vi "te.vi"() -> ()   [LabVIEW 2018]
uses:
  te_state.ctl
  Epimedia_Connex_Source/Controls/Enums/LogLoopEnum.ctl
  Epimedia_Connex_Source/Controls/Clusts/TE_Data_Clust.ctl
panel:
  out "ElapsedRead":u32
  out "Error Out":errorcluster
  out "Enum":T1
  out "Read Progress":dbl(slide) scale=0.0..1.0
  out "On? 3":dbl format="%#.0g"
  out "P 3":dbl format="%.2g"
  out "I 3":dbl format="%.2g"
  out "D 3":dbl format="%.2g"
  out "Set Point 3":dbl format="%.2g"
  out "Temp 3":dbl format="%.2g"
  out "Output 3":dbl format="%.2f"
  out "Polarity 3":dbl format="%#_1g"
  out "Control Type 3":dbl format="%#_1g"
  out "On? 2":dbl format="%#.0g"
  out "P 2":dbl format="%.2g"
  out "I 2":dbl format="%.2g"
  out "D 2":dbl format="%.2g"
  out "Set Point 2":dbl format="%.2g"
  out "Temp 2":dbl format="%.2g"
  out "Output 2":dbl format="%.2f"
  out "Polarity 2":dbl format="%#_1g"
  out "Control Type 2":dbl format="%#_1g"
  out "On?":dbl format="%#.0g"
  out "P 4":dbl format="%.2g"
  out "I 4":dbl format="%.2g"
  out "D 4":dbl format="%.2g"
  out "Set Point 4":dbl format="%.2g"
  out "Temp":dbl format="%.2g"
  out "Output":dbl format="%.2f"
  out "Polarity 4":dbl format="%#_1g"
  out "Control Type 4":dbl format="%#_1g"
  in  "On?":i32 min=0 max=1 format="%_1f"
  in  "P":dbl=5.0 format="%.2g"
  in  "I":dbl format="%.2g"
  in  "D":dbl format="%.2g"
  in  "Set Point":dbl=40.0 format="%.2g"
  in  "Control Type":i32=1 min=0 max=2 format="%_1f"
  in  "Polarity":i32 min=0 max=1 format="%_1f"
  in  "WriteAddressSelect":enum32{"Air", "Bottom Plate ", "Front Plate"}(radio)
  out "Header":picture
  in  "Address":string[](array[string])=["01", "02", "03"]
  in  "Port":refnum<visa-resource-name>="Port1"
  in  "Save Parameters":bool
  out "LED":bool
  in  "stop":bool
  out "Error Dialog":string="Error Message Display Box"
  out "Waveform Chart":cluster{"[0]":dbl, "[0]":dbl, "[0]":dbl}(graph)
  # "°C"
  # "Temp."
  # "%"
  # "Output"
  # "°C"
  # "Control Type:"
  # "0   Deadband\n1   PID\n2   Computer"
  # "Polarity:"
  # "0   HEAT WP1+ and WP2-\n1   HEAT WP2+ and WP1-"
  # "Original Creator: \nMike Zemba, NASA Glenn Research Center\nmichael.j.zemba@nasa.gov\nModified by:\nLuke Graham, Epimedia, Inc.\nluke@epimedia.com"
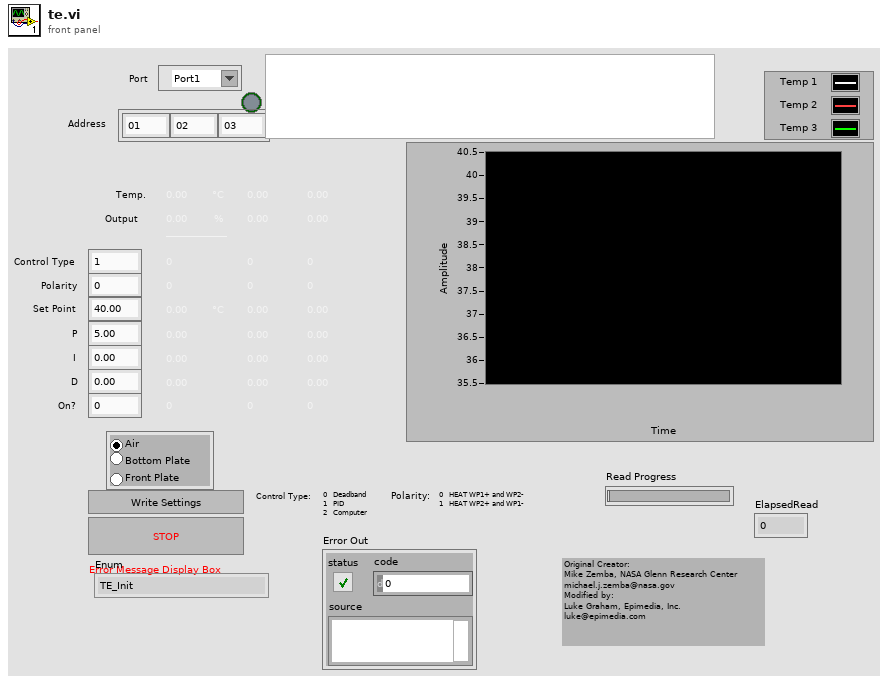
[diagram p1: front panel]
types:
  T1 = typedef "te_state.ctl" = enum16{"TE_Init", "TE_Autotune", "TE_Wait", "TE_Read", "TE_Display", "TE_Send", "TE_Write"}
  T2 = cluster{"port":refnum<visa-resource-name>, "timeout":u32, "baud":u32, "dataBits":u16, "stopBits":u16, "flowControl":u16, "parity":u16, "termChar":bool, "checkSum":bool, "checkSumVal":string}
  T3 = typedef "te_state.ctl" = enum16{"Config", "Autotune", "Wait", "Read", "Log"}
  T4 = typedef "TE_Data_Clust.ctl" = cluster{"TimeString":string, "TimeStamp":dbl, "Temp":dbl, "Output":dbl, "Temp 2":dbl, "Output 2":dbl, "Temp 3":dbl, "Output 3":dbl}
  T5 = typedef "LogLoopEnum.ctl" = enum16{"Log_Init", "Log_Config", "Log_CfgAlarm", "Log_TimeDomain", "Log_Tone", "Log_NoiseTrace", "Log_NoiseSum", "Log_DO", "Log_AI", "Log_TC", "Log_Disdrom", "Log_Weather", "Log_TE", "Log_ADAM", "Log_UPS", "Log_ChkTime", "Log_Alarm", "Log_Write", "Log_Exit"}
  T6 = typedef "imagedata.ctl" = cluster{"image type":i32, "image depth":i32, "image":u8[], "mask":u8[], "colors":u32[], "Rectangle":cluster{"left":i16, "top":i16, "right":i16, "bottom":i16}}
  T7 = cluster{"[0]":dbl, "[1]":dbl, "[2]":dbl, "[3]":dbl, "[4]":dbl, "[5]":dbl, "[6]":dbl, "[7]":dbl, "[8]":dbl}
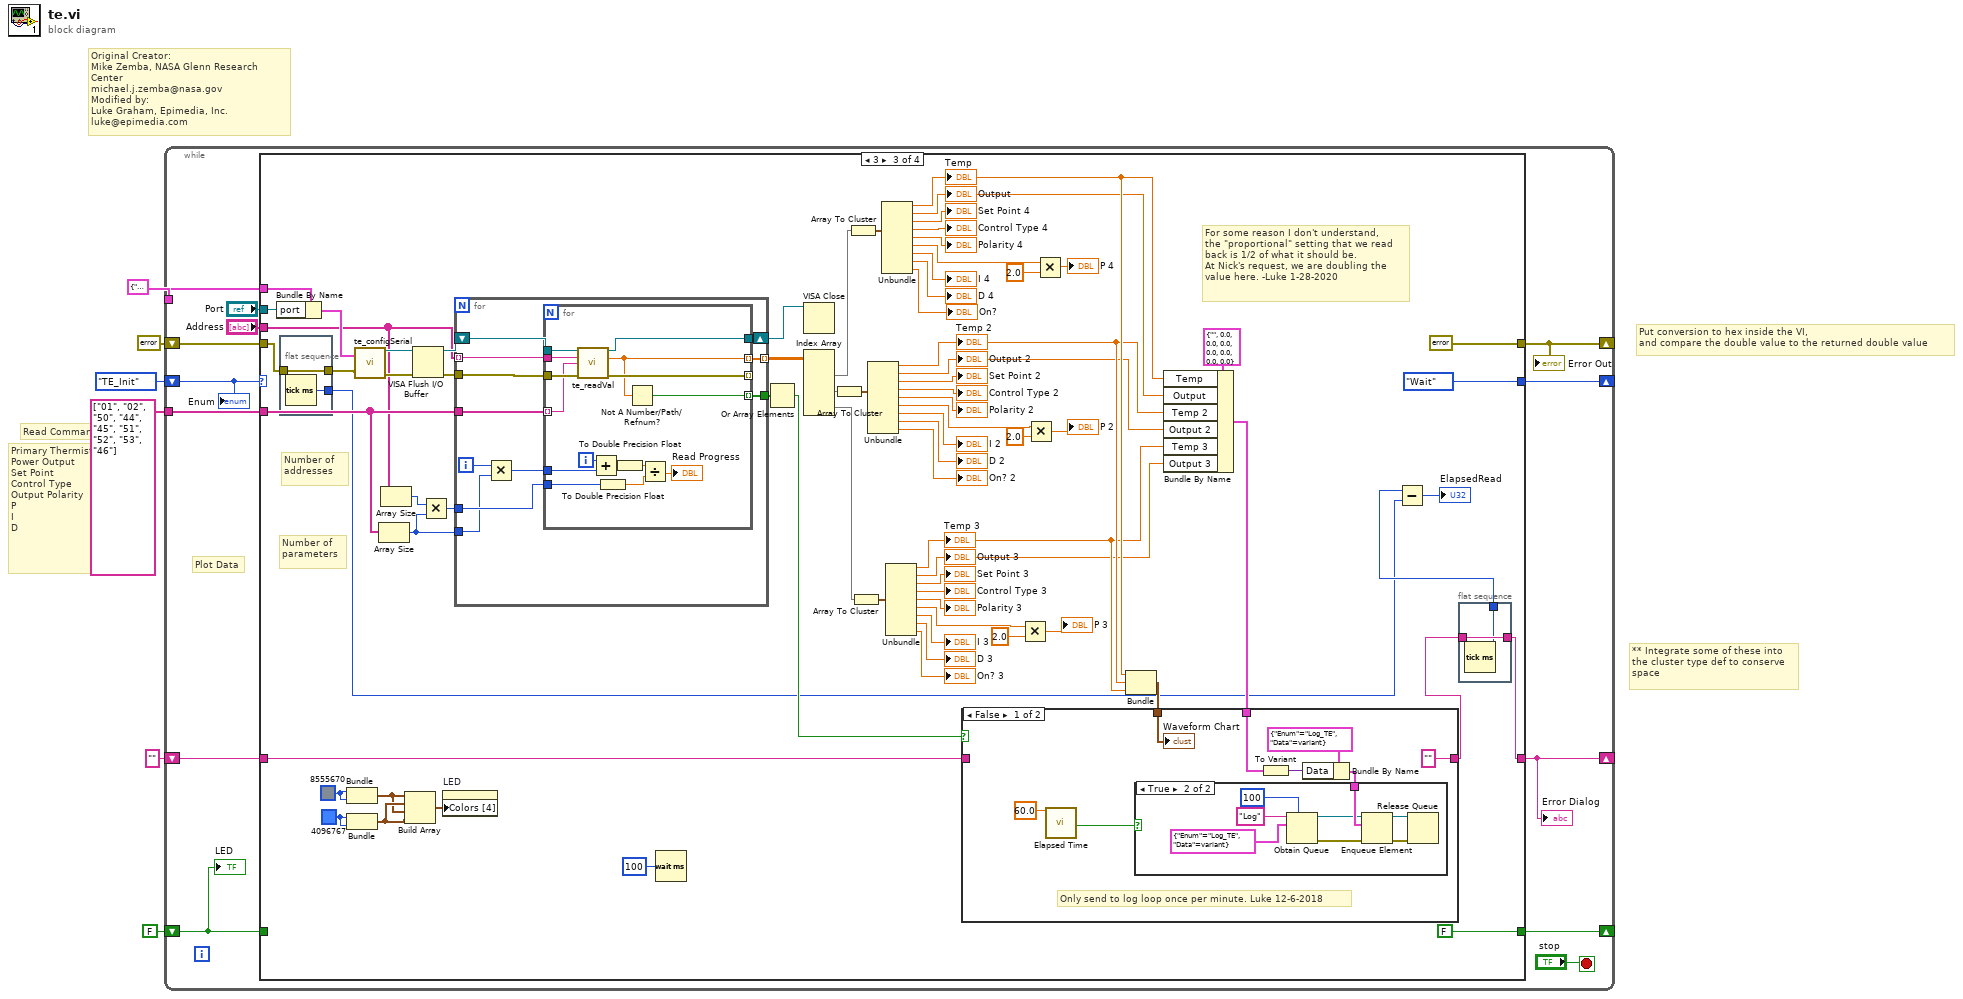
[diagram p0: block diagram]
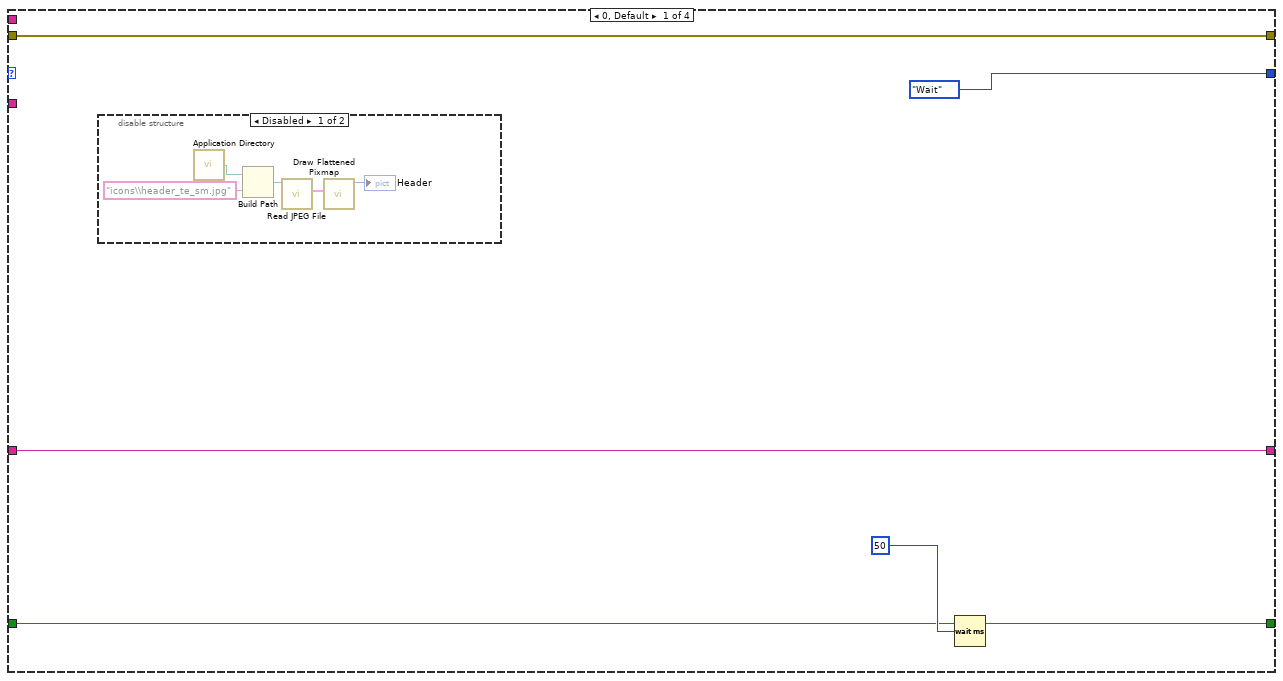
[diagram p2: hidden frame]
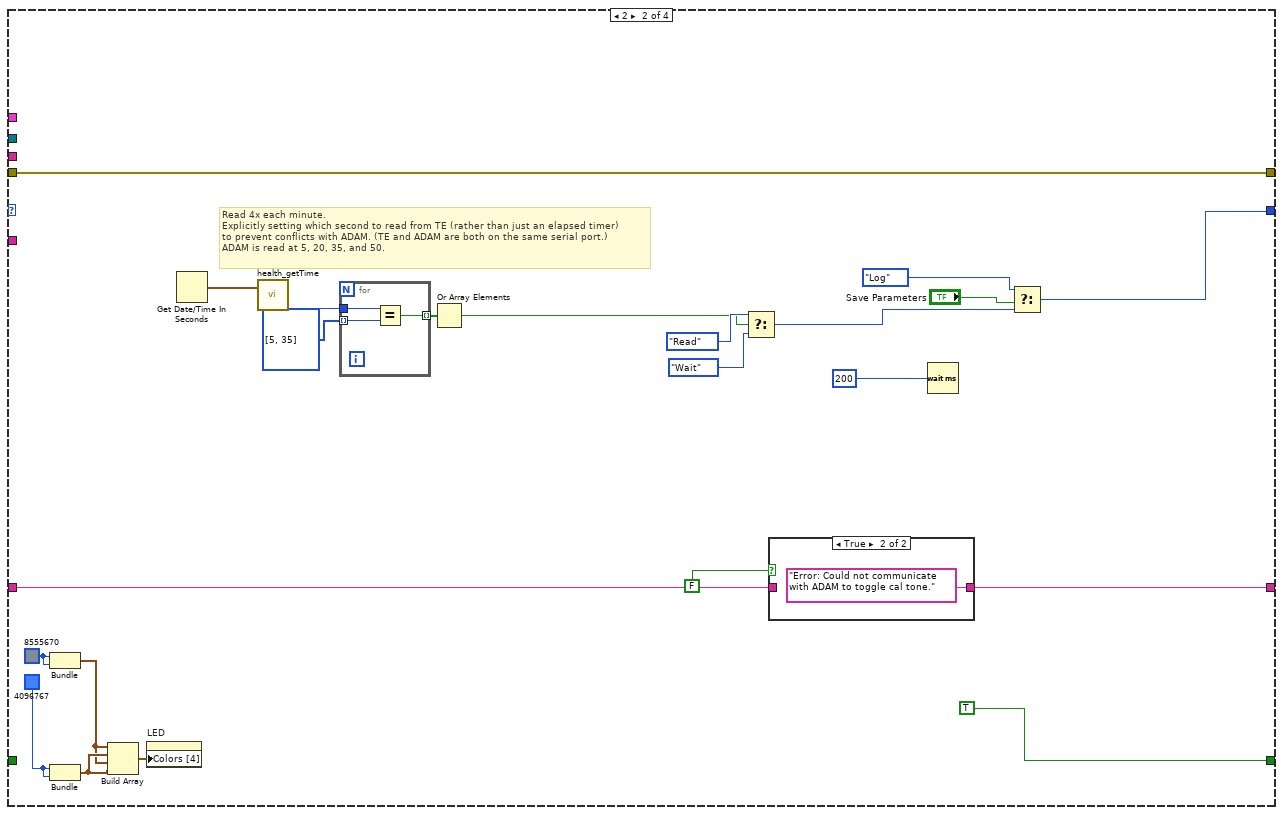
[diagram p4: hidden frame]
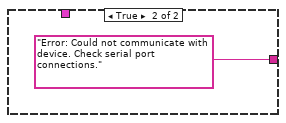
[diagram p7: hidden frame]
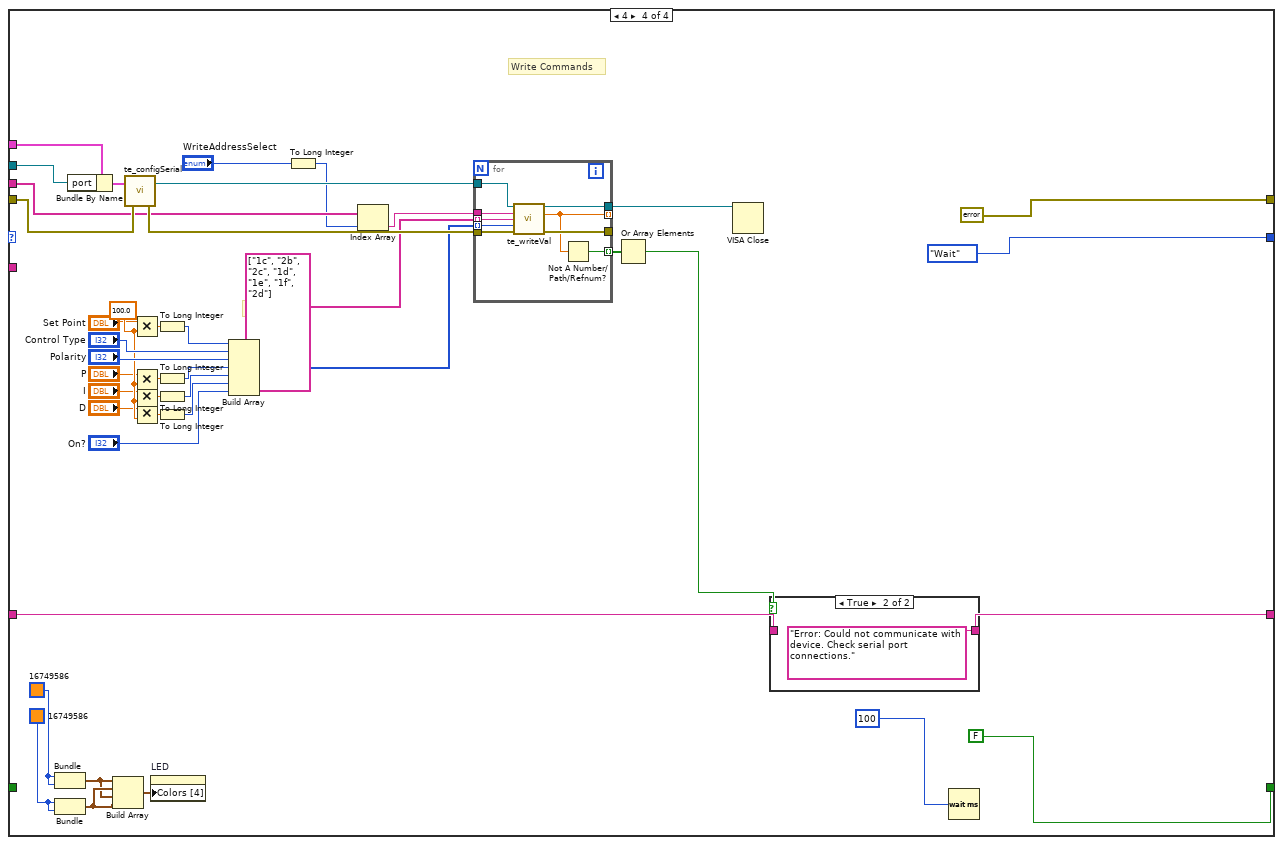
[diagram p8: hidden frame]
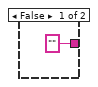
[diagram p9: hidden frame]
diagram:
  # "Original Creator: \nMike Zemba, NASA Glenn Research Center\nmichael.j.zemba@nasa.gov\nModified by:\nLuke Graham, Epimedia, Inc.\nluke@epimedia.com"
  # "Put conversion to hex inside the VI,\nand compare the double value to the returned double value"
  # "Read Commands"
  # "Primary Thermistor\nPower Output\nSet Point\nControl Type\nOutput Polarity\nP\nI\nD"
  # "** Integrate some of these into\nthe cluster type def to conserve\nspace"
  n1 = while {
    shift-right: [w18] -> _
    shift-left: te_state."TE_Init" ("Enum") -> [w19]
    shift-right: [w12] -> _
    shift-left: errorcluster {"status"=FALSE, "code"=0, "source"=""} ("Error Out") -> [w17]
    shift-right: [w16] -> _
    shift-left: FALSE -> [w7]
    shift-right: [w14] -> _
    shift-left: "" ("Error Dialog") -> [w13]
    tunnel: T2 {"port"="COM1", "timeout"=4000, "baud"=115200, "dataBits"=8, "stopBits"=10, "flowControl"=0, "parity"=0, "termChar"=FALSE, "checkSum"=FALSE, "checkSumVal"=""} ("teSerial") -> [w11]
    tunnel: string[] ["01", "02", "50", "44", "45", "51", "52", "53", "46"] -> [w10]
    stop <- "stop" stop-if-true
    # "Plot Data"
    n2 = case shown="3" w19 {
      tunnel: [te_state."Wait" ("Enum") w35 te_state."Wait" ("Enum") te_state."Wait" ("Enum")] -> w18
      tunnel: w17 -> [w20 w46 w70 w204]
      tunnel: [w22 TRUE FALSE FALSE] -> w16
      tunnel: w7 -> [w22 _ _ _]
      tunnel: [w21 w45 w68 w213] -> w14
      tunnel: w13 -> [w21 w44 w122 w211]
      tunnel: [w20 w46 errorcluster {"status"=FALSE, "code"=0, "source"=""} ("Error Out") errorcluster {"status"=FALSE, "code"=0, "source"=""} ("Error Out")] -> w12
      tunnel: w11 -> [_ _ w120 w209]
      tunnel: w10 -> [_ _ w84 _]
      tunnel: "Port" -> [_ _ w112 w208]
      tunnel: "Address" -> [_ _ w83 w183]
      frame 0, Default {
        n3 = disable-structure shown="Disabled" {
          frame Disabled {
            n4 = call <vilib>:"Application Directory.vi"() -> ("Application Directory"=w26:path)
            n5 = Build Path(base path=w26, name or relative path="icons\\header_te_sm.jpg") -> (appended path=w27:path)
            n6 = call <vilib>:"Read JPEG File.vi"("path to JPEG file"=w27) -> ("image data"=w29:T6)  [unwired: 8 in, 2 out]
            n7 = call <vilib>:"Draw Flattened Pixmap.vi"("image data"=w29) -> ("new picture"=→"Header":picture)  [unwired: 8 in]
          }
          frame Enabled {
          }
        }
        n8 = Wait (ms)(milliseconds to wait=u32 50) -> ()  [unwired: 1 out]
      }
      frame 2 {
        w50 = u32 4096767
        w49 = u32 8555670
        # "Read 4x each minute.\nExplicitly setting which second to read from TE (rather than just an elapsed timer)\nto prevent conflicts with ADAM. (TE and ADAM are both on the same serial port.)\nADAM is read at 5, 20, 35, and 50."
        n9 = Bundle(w49, w49) -> (w47:cluster{u32, u32})  [unwired: 1 in]
        n10 = Bundle(w50, w50) -> (w48:cluster{u32, u32})  [unwired: 1 in]
        n11 = Build Array(w47, w48, w47, w48) -> (w51:cluster{u32, u32}[])
        n12 = property on="LED" class="Bool (strict)"("Colors [4]"=w51) -> ()  [unwired: 2 in, 2 out]
        n13 = Get Date/Time In Seconds() -> (seconds since 1Jan1904=w30:timestamp)
        n14 = call "health_getTime.vi"("Current Time"=w30) -> ("Seconds"=w34:u32)  [unwired: 11 in, 7 out]
        n15 = for {
          tunnel: w34 -> [w54]
          tunnel: u32[] [5, 35] ("y") -> [w53] mode=indexing
          tunnel: [w52] -> w32 mode=indexing
          n16 = Equal?(x=w54, y=w53) -> (x = y?=w52:bool)
        }
        n17 = Or Array Elements(Boolean array=w32) -> (logical OR=w31:bool)
        n18 = Select(t=te_state."Read" ("Enum"), s=w31, f=te_state."Wait" ("Enum")) -> (s? t:f=w37:T3)
        n19 = case shown="True" FALSE {
          tunnel: [w55 "Error: Could not communicate with ADAM to toggle cal tone." ("Error Dialog")] -> w45
          tunnel: w44 -> [w55 _]
          frame False {
          }
          frame True {
          }
        }
        n20 = Wait (ms)(milliseconds to wait=u32 200 ("y")) -> ()  [unwired: 1 out]
        n21 = Select(t=te_state."Log" ("Enum"), s="Save Parameters", f=w37) -> (s? t:f=w35:T3)
      }
      frame 3 {
        w130 = u32 4096767
        w129 = u32 8555670
        # "For some reason I don't understand, \nthe \"proportional\" setting that we read\nback is 1/2 of what it should be.\nAt Nick's request, we are doubling the \nvalue here. -Luke 1-28-2020"
        # "Number of parameters"
        # "Number of addresses"
        n22 = Bundle By Name(cluster=w120, "port"=w112) -> (w111:T2)
        n23 = flat-sequence {
          tunnel: [w135] -> w71
          tunnel: w70 -> [w135]
          tunnel: [w134] -> w66
          frame #0 {
            n24 = Tick Count (ms)() -> (millisecond timer value=w134:u32)
          }
        }
        n25 = Bundle(w129, w129) -> (w127:cluster{u32, u32})  [unwired: 1 in]
        n26 = Bundle(w130, w130) -> (w128:cluster{u32, u32})  [unwired: 1 in]
        n27 = call "te_configSerial.vi"("Error In"=w71, "teSerial"=w111) -> ("error out"=w105:errorcluster, "VISA resource name out"=w107:refnum<visa-resource-name>)
        n28 = Array Size(array=w84) -> (size(s)=w80:i32)
        n29 = Array Size(array=w83) -> (size(s)=w81:i32)
        n30 = Build Array(w127, w128, w127, w128) -> (w125:cluster{u32, u32}[])
        n31 = VISA Flush I/O Buffer(VISA resource name=w107, error in (no error)=w105) -> (VISA resource name out=w106:refnum<visa-resource-name>, error out=w104:errorcluster)  [unwired: 1 in]
        n32 = Multiply(x=w81, y=w80) -> (x*y=w82:i32)
        n33 = property on="LED" class="Bool (strict)"("Colors [4]"=w125) -> ()  [unwired: 2 in, 2 out]
        n34 = for {
          tunnel: [w146] -> w124
          tunnel: w84 -> [w145]
          tunnel: [w144] -> w103 mode=indexing
          tunnel: w104 -> [w141]
          tunnel: w83 -> [w140] mode=indexing
          shift-right: [w143] -> w110
          shift-left: w106 -> [w142]
          tunnel: w82 -> [w138]
          tunnel: w80 -> [w136]
          i -> [w139]
          n35 = Multiply(x=w139, y=w136) -> (x*y=w137:i32)
          n36 = for {
            tunnel: [w156] -> w144 mode=indexing
            tunnel: w141 -> [w161]
            tunnel: [w160] -> w146 mode=indexing
            tunnel: [w159] -> _ mode=indexing
            tunnel: w140 -> [w158]
            tunnel: w145 -> [w157] mode=indexing
            tunnel: w142 -> [w155]
            tunnel: [w154] -> w143
            tunnel: w137 -> [w150]
            tunnel: w138 -> [w149]
            i -> [w153]
            n37 = call "te_readVal.vi"("VISA In"=w155, "Hex Address"=w158, "Command"=w157, "Error In"=w161) -> ("VISA Out"=w154:refnum<visa-resource-name>, "Response"=w156:dbl, "error out"=w159:errorcluster)  [unwired: 7 in, 2 out]
            n38 = Add(x=w153, y=w150) -> (x+y=w152:i32)
            n39 = To Double Precision Float(number=w149) -> (double precision float=w147:dbl)
            n40 = To Double Precision Float(number=w152) -> (double precision float=w148:dbl)
            n41 = Not A Number/Path/Refnum?(number/path/refnum=w156) -> (NaN/Path/Refnum?=w160:bool)
            n42 = Divide(x=w148, y=w147) -> (x/y=→"Read Progress":dbl)
          }
        }
        n43 = Wait (ms)(milliseconds to wait=u32 100) -> ()  [unwired: 1 out]
        n44 = Or Array Elements(Boolean array=w124) -> (logical OR=w123:bool)
        n45 = VISA Close(VISA resource name=w110) -> ()  [unwired: 1 in, 1 out]
        n46 = Index Array(array=w103) -> (element #1=w102:dbl[], element #2=w89:dbl[], element #3=w88:dbl[])  [unwired: 6 in]
        n47 = Array To Cluster(array=w89) -> (cluster=w101:T7)
        n48 = Array To Cluster(array=w102) -> (cluster=w119:T7)
        n49 = Array To Cluster(array=w88) -> (cluster=w90:T7)
        n50 = Unbundle(w101) -> ("[0]"=w77:dbl, "[1]"=w74:dbl, "[2]"=→"Set Point 2":dbl, "[3]"=→"Control Type 2":dbl, "[4]"=→"Polarity 2":dbl, "[5]"=w60:dbl, "[6]"=→"I 2":dbl, "[7]"=→"D 2":dbl, "[8]"=→"On? 2":dbl)
        "Temp 2" <- w77
        "Output 2" <- w74
        n51 = Unbundle(w119) -> ("[0]"=w78:dbl, "[1]"=w73:dbl, "[2]"=→"Set Point 4":dbl, "[3]"=→"Control Type 4":dbl, "[4]"=→"Polarity 4":dbl, "[5]"=w115:dbl, "[6]"=→"I 4":dbl, "[7]"=→"D 4":dbl, "[8]"=→"On?":dbl)
        "Temp" <- w78
        "Output" <- w73
        n52 = Unbundle(w90) -> ("[0]"=w76:dbl, "[1]"=w75:dbl, "[2]"=→"Set Point 3":dbl, "[3]"=→"Control Type 3":dbl, "[4]"=→"Polarity 3":dbl, "[5]"=w58:dbl, "[6]"=→"I 3":dbl, "[7]"=→"D 3":dbl, "[8]"=→"On? 3":dbl)
        "Temp 3" <- w76
        "Output 3" <- w75
        n53 = Multiply(x=w58, y=2.0) -> (x*y=→"P 3":dbl)
        n54 = Multiply(x=w60, y=2.0) -> (x*y=→"P 2":dbl)
        n55 = Multiply(x=w115, y=2.0) -> (x*y=→"P 4":dbl)
        n56 = Bundle("[0]"=w78, "[0]"=w77, "[0]"=w76) -> (w108:cluster{"[0]":dbl, "[0]":dbl, "[0]":dbl})  [unwired: 1 in]
        n57 = Bundle By Name(cluster=T4 {"TimeString"="", "TimeStamp"=0.0, "Temp"=0.0, "Output"=0.0, "Temp 2"=0.0, "Output 2"=0.0, "Temp 3"=0.0, "Output 3"=0.0}, "Temp"=w78, "Output"=w73, "Temp 2"=w77, "Output 2"=w74, "Temp 3"=w76, "Output 3"=w75) -> (w72:T4)
        n58 = case shown="False" w123 {
          tunnel: ["" ("Error Dialog") "Error: Could not communicate with device. Check serial port connections." ("Error Dialog")] -> w69
          tunnel: w122 -> [_ _]
          tunnel: w108 -> [w168 _]
          tunnel: w72 -> [w164 _]
          frame False {
            # "Only send to log loop once per minute. Luke 12-6-2018"
            n59 = call "Elapsed Time"("Time Target (s)"=60.0) -> ("Time has Elapsed"=w162:bool)  [unwired: 11 in, 7 out]
            n60 = To Variant(anything=w164) -> (Variant=w165:variant)
            n61 = Bundle By Name(cluster=cluster{"Enum":T5, "Data":variant} {"Enum"=enum."Log_TE", "Data"=variant}, "Data"=w165) -> (w167:cluster{"Enum":T5, "Data":variant})
            n62 = case shown="True" w162 {
              tunnel: w167 -> [_ w174]
              frame False {
              }
              frame True {
                n63 = Obtain Queue(max queue size (-1, unlimited)=100, name (unnamed)="Log", element data type=cluster{"Enum":T5, "Data":variant} {"Enum"=enum."Log_TE", "Data"=variant}) -> (queue out=w172:refnum<queue>, error out=w173:errorcluster)  [unwired: 2 in, 1 out]
                n64 = Enqueue Element(queue=w172, element=w174, error in (no error)=w173) -> (queue out=w175:refnum<queue>, error out=w176:errorcluster)  [unwired: 1 in, 1 out]
                n65 = Release Queue(queue=w175, error in (no error)=w176) -> ()  [unwired: 1 in, 3 out]
              }
            }
            "Waveform Chart" <- w168
          }
          frame True {
          }
        }
        n66 = Subtract(x=w67, y=w66) -> (x-y=→"ElapsedRead":u32)
        n67 = flat-sequence {
          tunnel: [w133] -> w68
          tunnel: w69 -> [w133]
          tunnel: [w132] -> w67
          frame #0 {
            n68 = Tick Count (ms)() -> (millisecond timer value=w132:u32)
          }
        }
      }
      frame 4 {
        w191 = 100.0 ("y")
        w219 = u32 16749586
        w218 = u32 16749586
        # "Set Data"
        # "Write Commands"
        n69 = Bundle(w218, w218) -> (w216:cluster{u32, u32})  [unwired: 1 in]
        n70 = Bundle(w219, w219) -> (w217:cluster{u32, u32})  [unwired: 1 in]
        n71 = Bundle By Name(cluster=w209, "port"=w208) -> (w206:T2)
        n72 = Build Array(w216, w217, w216, w217) -> (w215:cluster{u32, u32}[])
        n73 = call "te_configSerial.vi"("Error In"=w204, "teSerial"=w206) -> ("error out"=w205:errorcluster, "VISA resource name out"=w207:refnum<visa-resource-name>)
        n74 = Multiply(x="Set Point", y=w191) -> (x*y=w192:dbl)
        n75 = Multiply(x="P", y=w191) -> (x*y=w195:dbl)
        n76 = Multiply(x="I", y=w191) -> (x*y=w194:dbl)
        n77 = Multiply(x="D", y=w191) -> (x*y=w193:dbl)
        n78 = property on="LED" class="Bool (strict)"("Colors [4]"=w215) -> ()  [unwired: 2 in, 2 out]
        n79 = To Long Integer(number=w192) -> (32bit integer=w196:i32)
        n80 = To Long Integer(number=w195) -> (32bit integer=w199:i32)
        n81 = To Long Integer(number=w194) -> (32bit integer=w200:i32)
        n82 = To Long Integer(number=w193) -> (32bit integer=w201:i32)
        n83 = Build Array(w196, "Control Type", "Polarity", w199, w200, w201, "On?") -> (w186:i32[])
        n84 = To Long Integer(number="WriteAddressSelect") -> (32bit integer=w180:i32)
        n85 = Index Array(array=w183, index=w180) -> (element=w182:string)
        n86 = for {
          tunnel: [w226] -> _ mode=indexing
          tunnel: w205 -> [w231]
          tunnel: [w230] -> w214 mode=indexing
          tunnel: [w229] -> _
          tunnel: w182 -> [w228]
          tunnel: string[] ["1c", "2b", "2c", "1d", "1e", "1f", "2d"] -> [w227] mode=indexing
          tunnel: w207 -> [w225]
          tunnel: [w224] -> w203
          tunnel: w186 -> [w223] mode=indexing
          n87 = call "te_writeVal.vi"("VISA In"=w225, "Hex Address"=w228, "Command"=w227, "Data"=w223, "Error In"=w231) -> ("VISA Out"=w224:refnum<visa-resource-name>, "Response"=w226:dbl, "error out"=w229:errorcluster)  [unwired: 7 in, 1 out]
          n88 = Not A Number/Path/Refnum?(number/path/refnum=w226) -> (NaN/Path/Refnum?=w230:bool)
        }
        n89 = Or Array Elements(Boolean array=w214) -> (logical OR=w212:bool)
        n90 = VISA Close(VISA resource name=w203) -> ()  [unwired: 1 in, 1 out]
        n91 = case shown="True" w212 {
          tunnel: ["" ("Error Dialog") "Error: Could not communicate with device. Check serial port connections." ("Error Dialog")] -> w213
          tunnel: w211 -> [_ _]
          frame False {
          }
          frame True {
          }
        }
        n92 = Wait (ms)(milliseconds to wait=u32 100) -> ()  [unwired: 1 out]
      }
    }
    "Error Dialog" <- w14
    "Error Out" <- w12
    "LED" <- w7
    "Enum" <- w19
  }
